vi "lB 2.vi"() -> ()   [LabVIEW 2020]
panel:
  out "Sorted array":dbl[](array[numeric])
  out "Unsorted Array":dbl[](array[numeric])
  in  "Numeric":dbl
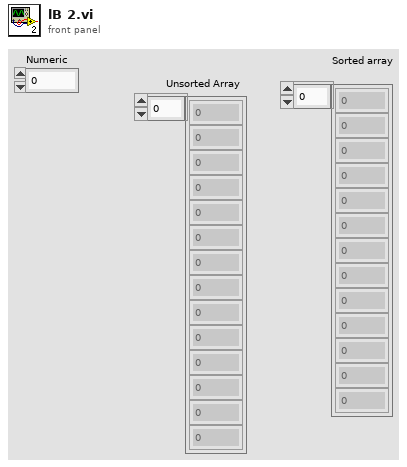
[diagram p1: front panel]
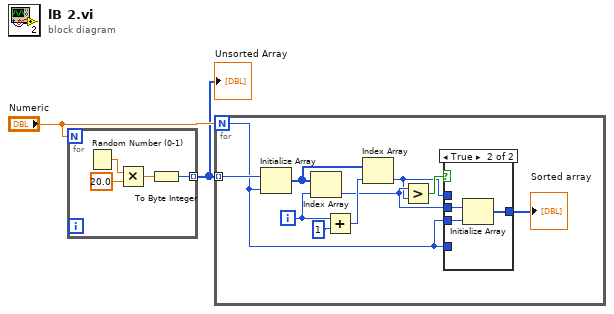
[diagram p0: block diagram]
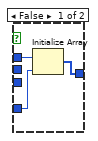
[diagram p2: hidden frame]
diagram:
  n1 = for {
    N: "Numeric" -> [_]
    tunnel: [w4] -> w1 mode=indexing
    n2 = Random Number (0-1)() -> (number: 0 to 1=w6:dbl)
    n3 = Multiply(x=w6, y=20.0) -> (x*y=w5:dbl)
    n4 = To Byte Integer(number=w5) -> (8bit integer=w4:i8)
  }
  "Unsorted Array" <- w1
  n5 = for {
    N: "Numeric" -> [w8]
    tunnel: w1 -> [w16] mode=indexing
    i -> [w14]
    n6 = Initialize Array(w16, w8) -> (w12:i8[])
    n7 = Index Array(array=w12, index=w14) -> (element=w10:i8)
    n8 = Add(x=w14, y=1) -> (x+y=w15:i32)
    n9 = Index Array(array=w12, index=w15) -> (element=w7:i8)
    n10 = Greater?(x=w10, y=w7) -> (0:w11:bool)
    n11 = case shown="True" w11 {
      tunnel: [w17 w22] -> w9
      tunnel: w10 -> [_ w20]
      tunnel: w8 -> [_ w21]
      tunnel: w8 -> [w19 _]
      tunnel: w7 -> [w18 _]
      frame False {
        n12 = Initialize Array(w18, w19) -> (w17:i8[])
      }
      frame True {
        n13 = Initialize Array(w20, w21) -> (w22:i8[])
      }
    }
    "Sorted array" <- w9
  }
